vi "Actor Core.vi"(8 "error in":errorcluster, 11 "BasicTerminalBinding In":refnum<class "BasicTerminalBinding.lvclass">) -> (0 "error out":errorcluster, 3 "Actor out":refnum<class "Actor.lvclass">)   [LabVIEW 2017, in "TestViewables.lvlib" / "BasicTerminalBinding.lvclass"]
doc: "(<B>Filename</B>: Actor Framework.lvlib:Actor.lvclass:Actor Core.vi)\n\nReceives messages to the actor, reacts to them, and initiates any error handling that may shut the actor down.\n\nDescendant classes may override this VI to append parallel tasks for the actor to complete while it handles messages. Overrides use the Call Parent Method node.\n\n<License>\nCopyright © 2017 Composed Systems, LLC | All rights reserved\nwww.composed.io\n\nAuthor: Ethan Stern <ethan.stern@composed.io>\n\nThis software is provided \"AS IS\" WITHOUT WARRANTIES, either express or implied, AND IS FOR EDUCATIONAL PURPOSES ONLY.\n</License>"
uses:
  BasicTerminalBinding.lvclass
  C:/Git/mva-framework/Framework/IViewable/IViewable/IViewable.lvclass
  <vilib>/ActorFramework/Actor/Actor.lvclass
  Framework/IViewable/IViewable/IViewable.lvclass
panel:
  out "Random Number":dbl format="%.3f"
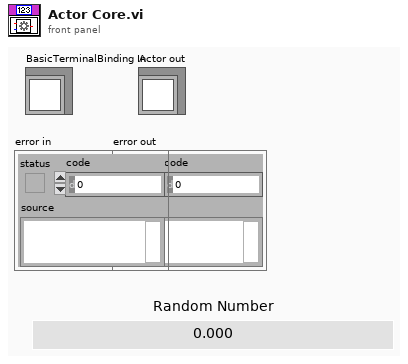
[diagram p1: front panel]
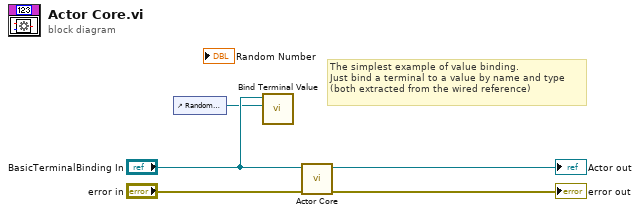
[diagram p0: block diagram]
diagram:
  # "The simplest example of value binding.\nJust bind a terminal to a value by name and type\n(both extracted from the wired reference)"
  n1 = control-ref of="Random Number"() -> (w1:refnum<vi>)
  n2 = call "Bind Terminal Value.vi"("Ctl Refnum"=w1, "IViewable in"="BasicTerminalBinding In") -> ()  [unwired: 8 in, 2 out]
  n3 = call-parent "Actor Core.vi"("error in"="error in", "IViewable In"="BasicTerminalBinding In") -> ("error out"=→"error out":errorcluster, "Actor out"=→"Actor out":refnum<class "Actor.lvclass">)  [unwired: 8 in]
